vi "gfitsio-check-image-for-write.vi"(4 "lpixel":i32[](array[numeric]), 6 "fpixel":i32[](array[numeric]), 8 "error in (no error)":errorcluster, 11 "gfits refnum":T1) -> (0 "error out":errorcluster, 3 "dup gfits refnum":T1)   [LabVIEW 2013, in "gfitsio.lvlib"]
doc: "Check the input parameters against the image. If there is a mismatch in dimensionality or if a parameter is out of range for the image return an error."
uses:
  gfitsio.lvlib
  gfitsio-refnum.ctl
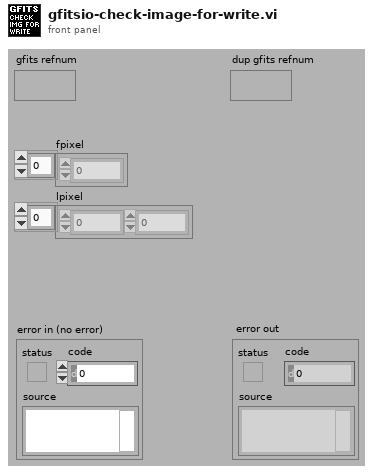
[diagram p1: front panel]
types:
  T1 = typedef "gfitsio.lvlib/gfitsio-refnum.ctl" = refnum<k1>
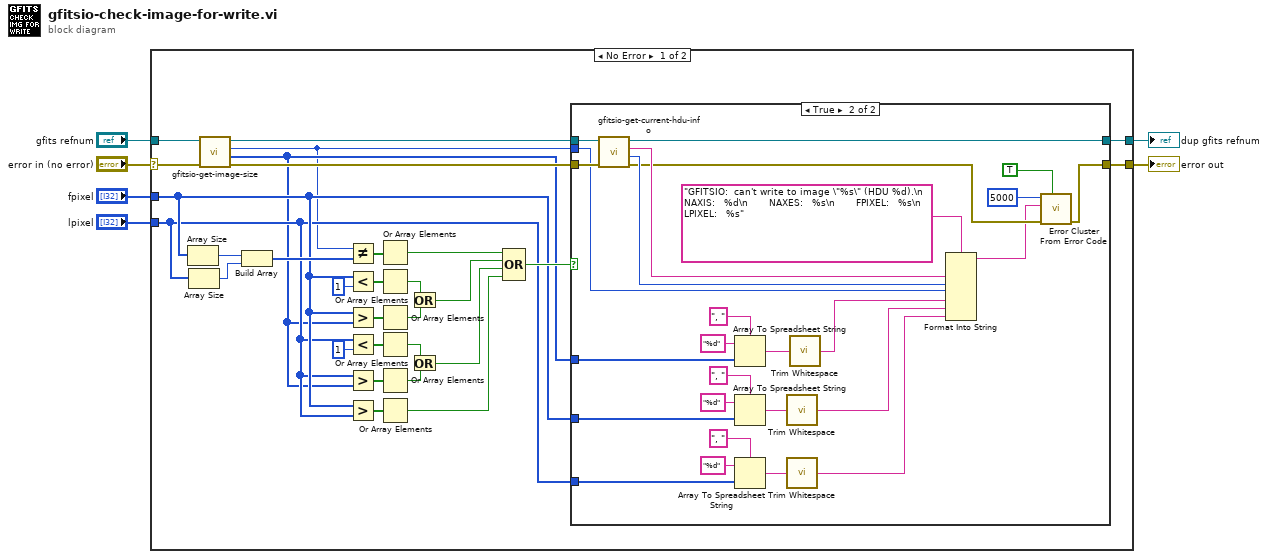
[diagram p0: block diagram]
diagram:
  n1 = case shown="No Error" "error in (no error)" {
    selector: "error in (no error)" -> [w11 w67]
    tunnel: "gfits refnum" -> [w12 w66]
    tunnel: [w21 w66] -> w2
    tunnel: "fpixel" -> [w14 _]
    tunnel: "lpixel" -> [w13 _]
    tunnel: [w16 w67] -> w1
    frame No Error {
      n2 = Array Size(array=w14) -> (size(s)=w25:i32)
      n3 = Array Size(array=w13) -> (size(s)=w24:i32)
      n4 = call "gfitsio-get-image-size.vi"("error in (no error)"=w11, "gfits refnum"=w12) -> ("error out"=w9:errorcluster, "naxes"=w8:i32[], "naxis"=w7:i32, "dup gfits refnum"=w10:T1)  [unwired: 6 out]
      n5 = Build Array(w25, w24) -> (w23:i32[])
      n6 = Not Equal?(x=w7, y=w23) -> (x != y?=w22:bool[])
      n7 = Less?(x=w14, y=1 ("x")) -> (x < y?=w35:bool[])
      n8 = Greater?(x=w14, y=w8) -> (0:w34:bool[])
      n9 = Less?(x=w13, y=1 ("x")) -> (x < y?=w28:bool[])
      n10 = Greater?(x=w13, y=w8) -> (0:w29:bool[])
      n11 = Greater?(x=w14, y=w13) -> (0:w26:bool[])
      n12 = Or Array Elements(Boolean array=w22) -> (logical OR=w20:bool)
      n13 = Or Array Elements(Boolean array=w35) -> (logical OR=w33:bool)
      n14 = Or Array Elements(Boolean array=w34) -> (logical OR=w32:bool)
      n15 = Or Array Elements(Boolean array=w28) -> (logical OR=w30:bool)
      n16 = Or Array Elements(Boolean array=w29) -> (logical OR=w31:bool)
      n17 = Or Array Elements(Boolean array=w26) -> (logical OR=w17:bool)
      n18 = Or(x=w33, y=w32) -> (x .or. y?=w19:bool)
      n19 = Or(x=w30, y=w31) -> (x .or. y?=w18:bool)
      n20 = Compound Arithmetic op=OR(w20, w19, w18, w17) -> (w15:bool)
      n21 = case shown="True" w15 {
        tunnel: w10 -> [w38 w65]
        tunnel: w9 -> [w37 w64]
        tunnel: [w37 w42] -> w16
        tunnel: [w38 w63] -> w21
        tunnel: w7 -> [_ w47]
        tunnel: w8 -> [_ w46]
        tunnel: w14 -> [_ w45]
        tunnel: w13 -> [_ w44]
        frame False {
        }
        frame True {
          n22 = call "gfitsio-get-current-hdu-info.vi"("error in (no error)"=w64, "gfits refnum"=w65) -> ("error out"=w43:errorcluster, "hdu number"=w48:i32, "hdu name"=w49:string, "dup gfits refnum"=w63:T1)  [unwired: 5 in, 1 out]
          n23 = Array To Spreadsheet String(delimiter (Tab)=", ", array=w46, 3:"%d" ("format string")) -> (spreadsheet string=w54:string)
          n24 = Array To Spreadsheet String(delimiter (Tab)=", ", array=w45, 3:"%d" ("format string")) -> (spreadsheet string=w60:string)
          n25 = Array To Spreadsheet String(delimiter (Tab)=", ", array=w44, 3:"%d" ("format string")) -> (spreadsheet string=w53:string)
          n26 = call <vilib>:"Trim Whitespace.vi"("string"=w60) -> ("trimmed string"=w51:string)  [unwired: 1 in]
          n27 = call <vilib>:"Trim Whitespace.vi"("string"=w53) -> ("trimmed string"=w52:string)  [unwired: 1 in]
          n28 = call <vilib>:"Trim Whitespace.vi"("string"=w54) -> ("trimmed string"=w50:string)  [unwired: 1 in]
          n29 = Format Into String(format string="GFITSIO:  can't write to image \"%s\" (HDU %d).\n       NAXIS:   %d\n       NAXES:   %s\n       FPIXEL:   %s\n       LPIXEL:   %s" ("error message (\"\")"), w49, w48, w47, w50, w51, w52) -> (resulting string=w39:string)  [unwired: 2 in, 1 out]
          n30 = call <vilib>:"Error Cluster From Error Code.vi"("show call chain? (False)"=TRUE, "error in (no error)"=w43, "error message (\"\")"=w39, "error code (0)"=5000) -> ("error out"=w42:errorcluster)  [unwired: 5 in]
        }
      }
    }
    frame Error {
    }
  }
  "error out" <- w1
  "dup gfits refnum" <- w2
